vi "ddr_read.vi"(5 "COM":bool, 7 "VISA name":refnum<visa-resource-name>, 10 "dwStartAddr":u32, 11 "dwLen":u32) -> (2 "pbydata":u8[](array[numeric]), 3 "return":i32)   [LabVIEW 2016]
panel:
  in  "tVdCmdHeader":T1
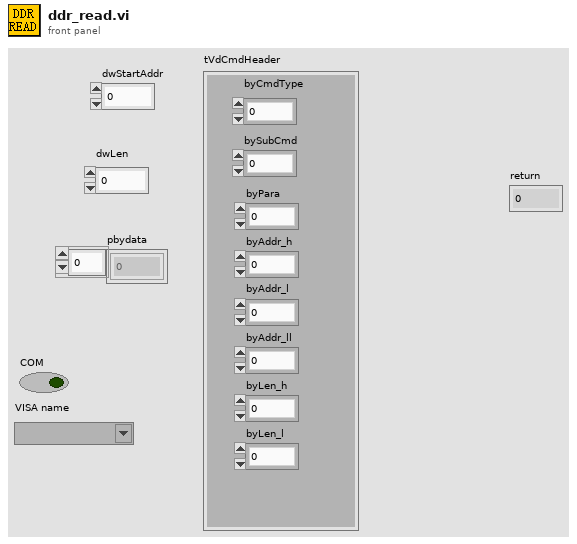
[diagram p1: front panel]
types:
  T1 = cluster{"byCmdType":u8, "bySubCmd":u8, "byPara":u8, "byAddr_h":u8, "byAddr_l":u8, "byAddr_ll":u8, "byLen_h ":u8, "byLen_l":u8}
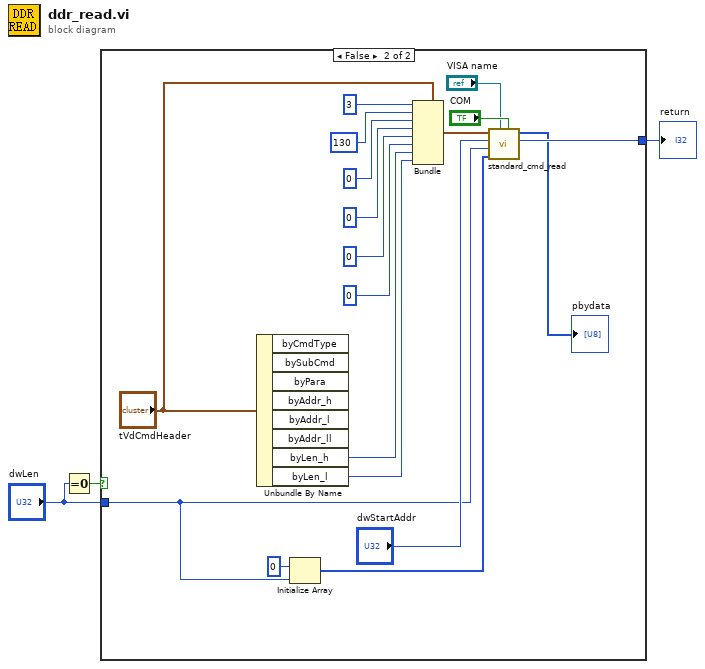
[diagram p0: block diagram]
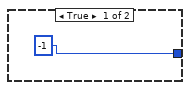
[diagram p2: hidden frame]
diagram:
  n1 = Equal To 0?(x="dwLen") -> (x = 0?=w2:bool)
  n2 = case shown="False" w2 {
    tunnel: [-1 w12] -> w3
    tunnel: "dwLen" -> [_ w5]
    frame True {
    }
    frame False {
      n3 = Unbundle By Name("tVdCmdHeader") -> ("byLen_h"=w19:u8, "byLen_l"=w18:u8)  [unwired: 6 out]
      n4 = Initialize Array(u8 0 ("element"), w5) -> (w7:u8[])
      n5 = Bundle(cluster="tVdCmdHeader", "byCmdType"=u8 3, "bySubCmd"=u8 130, "byPara"=u8 0, "byAddr_h"=u8 0, "byAddr_l"=u8 0, "byAddr_ll"=u8 0, "byLen_h"=w19, "byLen_l"=w18) -> (w17:T1)
      n6 = call "standard_cmd_read.vi"("COM"="COM", "VISA name"="VISA name", "data"=w7, "dwLen"=w5, "dwAddr"="dwStartAddr", "cmd_std_header_t"=w17) -> ("return"=w12:i32, "data out"=→"pbydata":u8[])  [unwired: 4 in]
    }
  }
  "return" <- w3
